vi "moveToLimit.vi"(2 "direction":i32, 3 "axis":i32, 4 "errorIn":errorcluster, 5 "referenceIn":refnum<k24>) -> (0 "errorOut":errorcluster, 1 "referenceOut":refnum<k24>)   [LabVIEW 2013]
uses:
  C:/Program Files/Newport/Piezo Motion Control/Newport AG-UC2-UC8 Applet/Samples/LabVIEW 2009/AgilisCmdLib.dll
  Program Files/Newport/Piezo Motion Control/Newport AG-UC2-UC8 Applet/Samples/LabVIEW 2009/AgilisCmdLib.dll
panel:
  # "Parameter \"direction\" must be either +1 (pos. direction) or -1 (neg. direction)."
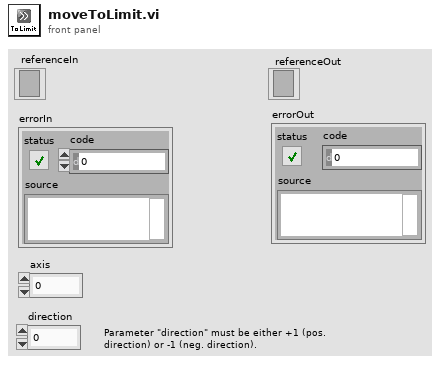
[diagram p1: front panel]
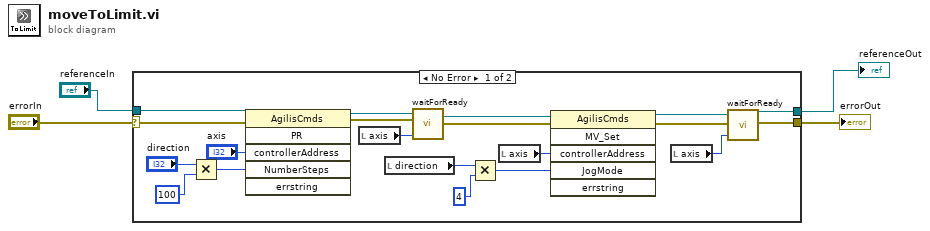
[diagram p0: block diagram]
diagram:
  n1 = case shown="No Error" "errorIn" {
    selector: "errorIn" -> [w22 w25]
    tunnel: "referenceIn" -> [w24 w26]
    tunnel: [w12 w26] -> w1
    tunnel: [w11 w25] -> w2
    frame No Error {
      n2 = Multiply(x="direction", y=100) -> (x*y=w19:i32)
      n3 = invoke class="AgilisCmds" method="PR"(reference=w24, error in=w22, "controllerAddress"="axis", "NumberSteps"=w19) -> (reference out=w9:refnum<k24>, error out=w7:errorcluster)  [unwired: 2 in, 4 out]
      n4 = local read "axis"() -> (w5:i32)
      n5 = local read "direction"() -> (w17:i32)
      n6 = call "waitForReady.vi"("axis"=w5, "errorIn"=w7, "referenceIn"=w9) -> ("errorOut"=w6:errorcluster, "referenceOut"=w8:refnum<k24>)
      n7 = Multiply(x=w17, y=4) -> (x*y=w16:i32)
      n8 = local read "axis"() -> (w18:i32)
      n9 = invoke class="AgilisCmds" method="MV_Set"(reference=w8, error in=w6, "controllerAddress"=w18, "JogMode"=w16) -> (reference out=w14:refnum<k24>, error out=w13:errorcluster)  [unwired: 2 in, 4 out]
      n10 = local read "axis"() -> (w10:i32)
      n11 = call "waitForReady.vi"("axis"=w10, "errorIn"=w13, "referenceIn"=w14) -> ("errorOut"=w11:errorcluster, "referenceOut"=w12:refnum<k24>)
    }
    frame Error {
    }
  }
  "referenceOut" <- w1
  "errorOut" <- w2
